vi "PV VOC Sensor Decode.vi"(11 "HEX Data (U8) in":u8[](array[numeric]) format="%x") -> (3 "VOC (kOhms)":string)   [LabVIEW 2023]
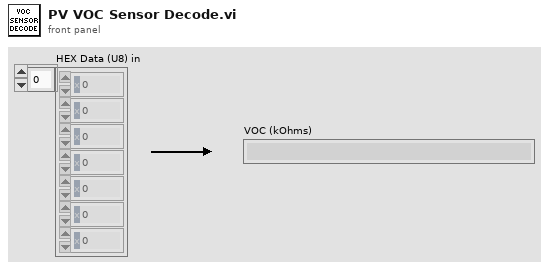
[diagram p1: front panel]
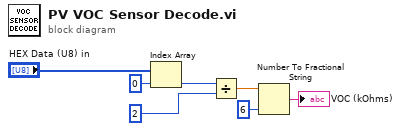
[diagram p0: block diagram]
diagram:
  n1 = Index Array(array="HEX Data (U8) in", index=0) -> (element=w5:u8)
  n2 = Divide(x=w5, y=u8 2) -> (x/y=w3:dbl)
  n3 = Number To Fractional String(number=w3, precision (6)=i16 6) -> (F-format string=→"VOC (kOhms)":string)  [unwired: 2 in]
